vi "SystemLog_with_Time.vi"(6 "SysLog_Queue":refnum<queue>, 7 "Message_in":string, 8 "error in (no error)":errorcluster, 9 "Send_Msg":string, 10 "Tick_in":dbl, 11 "Worker_Queue":refnum<queue>) -> (0 "error out":errorcluster)   [LabVIEW 2014]
uses:
  1005_GyuwonSourceProject/00_QMH_APIs/Gyu_Message_Data_Ctl.ctl
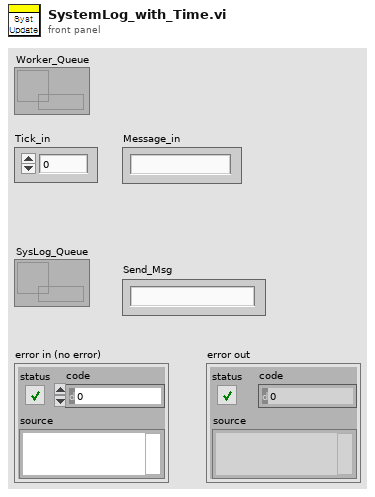
[diagram p1: front panel]
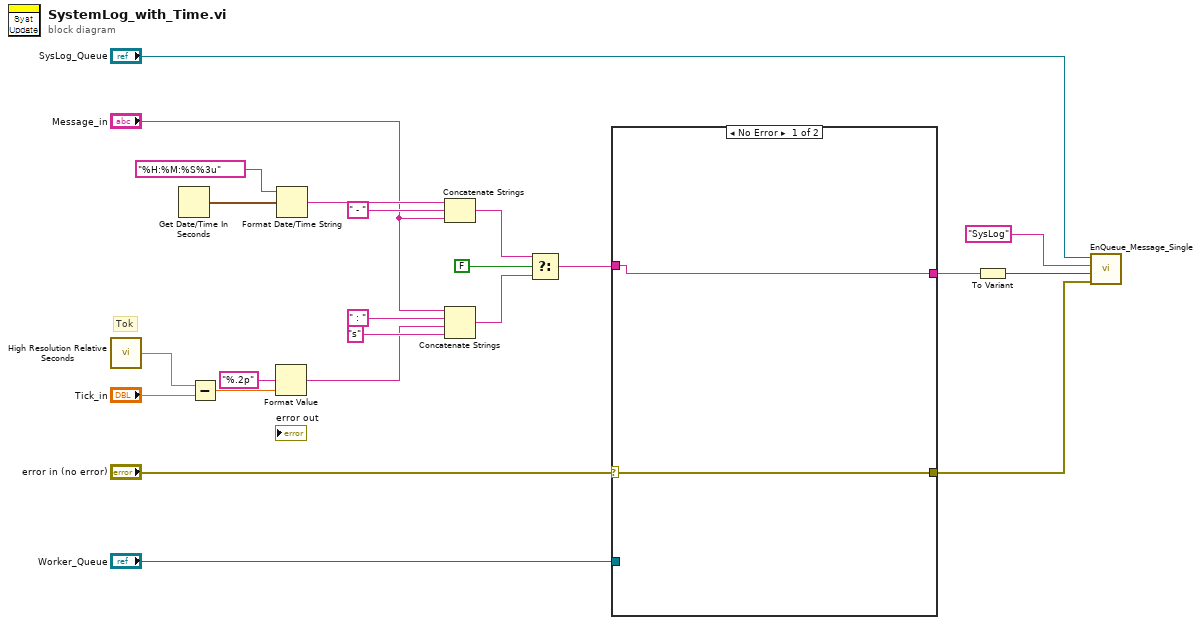
[diagram p0: block diagram]
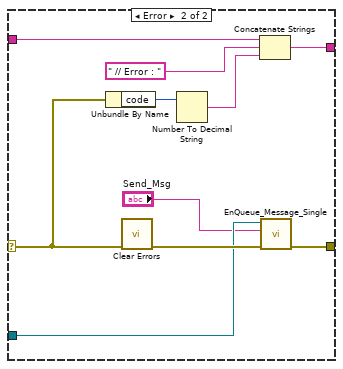
[diagram p2: hidden frame]
diagram:
  # "Tok"
  n1 = call <vilib>:"High Resolution Relative Seconds.vi"() -> ("relative seconds"=w22:dbl)
  n2 = Get Date/Time In Seconds() -> (seconds since 1Jan1904=w15:timestamp)
  n3 = Subtract(x=w22, y="Tick_in") -> (x-y=w20:dbl)
  n4 = Format Value(format string="%.2p", value (0)=w20) -> (output string=w17:string)  [unwired: 1 in]
  n5 = Format Date/Time String(time format string (%c)="%H:%M:%S%3u", seconds (now)=w15) -> (date/time string=w14:string)  [unwired: 1 in]
  n6 = Concatenate Strings(w14, " - ", "Message_in") -> (w10:string)
  n7 = Concatenate Strings("Message_in", " : ", w17, "s") -> (w11:string)
  n8 = Select(t=w10, s=FALSE, f=w11) -> (s? t:f=w7:string)
  n9 = case shown="No Error" "error in (no error)" {
    selector: "error in (no error)" -> [w24 w32]
    tunnel: w7 -> [w25 w31]
    tunnel: [w25 w30] -> w5
    tunnel: "Worker_Queue" -> [_ w27]
    tunnel: [w24 w28] -> w1
    frame No Error {
    }
    frame Error {
      n10 = Unbundle By Name(w32) -> ("code"=w35:i32)
      n11 = call <vilib>:"Clear Errors.vi"("error in (no error)"=w32) -> ("error out"=w29:errorcluster)  [unwired: 5 in, 1 out]
      n12 = Number To Decimal String(number=w35) -> (decimal integer string=w33:string)  [unwired: 1 in]
      n13 = Concatenate Strings(w31, " // Error : ", w33) -> (w30:string)
      n14 = call "EnQueue_Message_Single.vi"("error in (no error)"=w29, "Message"="Send_Msg", "Message_Queue"=w27) -> ("error out"=w28:errorcluster)  [unwired: 7 in, 1 out]
    }
  }
  n15 = To Variant(anything=w5) -> (Variant=w2:variant)
  n16 = call "EnQueue_Message_Single.vi"("error in (no error)"=w1, "Message Data"=w2, "Message"="SysLog", "Message_Queue"="SysLog_Queue") -> ()  [unwired: 6 in, 2 out]
